vi "Replace_data_in_setup_string.vi"(1 "New data string":string, 2 "Input string":string, 3 "Variable name":string) -> (0 "Appended string":string)   [LabVIEW 2020]
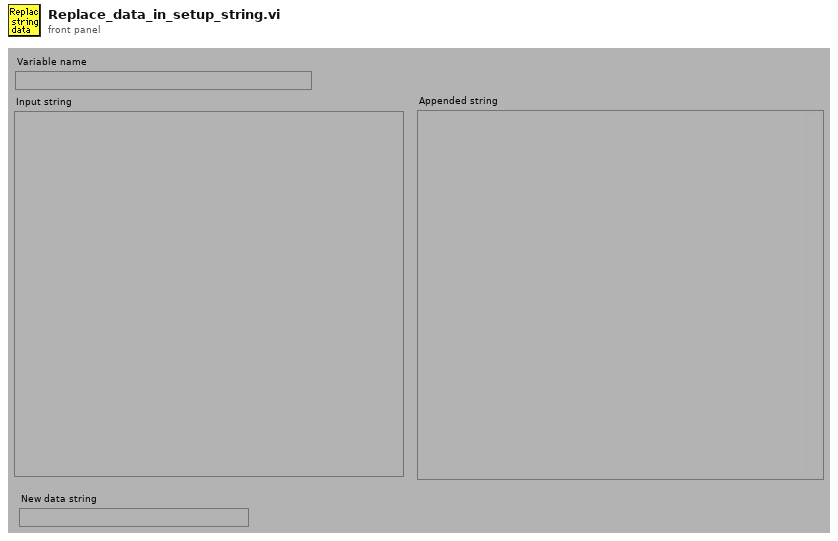
[diagram p1: front panel]
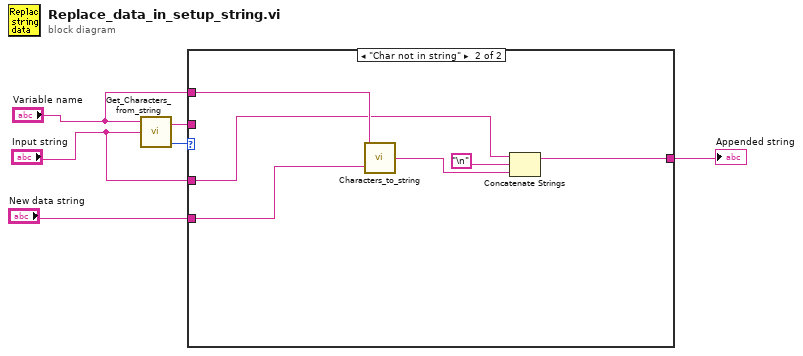
[diagram p0: block diagram]
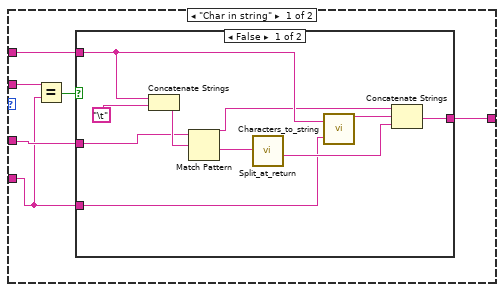
[diagram p2: hidden frame]
diagram:
  n1 = call "Get_Characters_from_string.vi"("Input string"="Input string", "Variable name"="Variable name") -> ("Status"=w6:enum16{"Char in string", "Char not in string"}, "Value"=w1:string)  [unwired: 1 in]
  n2 = case shown="\"Char not in string\"" w6 {
    tunnel: "Variable name" -> [w10 w29]
    tunnel: "New data string" -> [w8 w28]
    tunnel: [w11 w27] -> w3
    tunnel: "Input string" -> [w12 w26]
    tunnel: w1 -> [w9 _]
    frame "Char in string" {
      n3 = Equal?(x=w9, y=w8) -> (x = y?=w7:bool)
      n4 = case shown="False" w7 {
        tunnel: w12 -> [w20 w23]
        tunnel: [w17 w23] -> w11
        tunnel: w8 -> [w16 _]
        tunnel: w10 -> [w15 _]
        frame False {
          n5 = Concatenate Strings(w15, "\t") -> (w21:string)
          n6 = Match Pattern(string=w20, regular expression=w21) -> (before substring=w13:string, after substring=w19:string)  [unwired: 3 out]
          n7 = call "Split_at_return.vi"("String"=w19) -> ("after substring"=w18:string)  [unwired: 1 in, 3 out]
          n8 = call "Characters_to_string.vi"("Characters to write"=w16, "Label for characters"=w15) -> ("Output string"=w14:string)  [unwired: 1 in]
          n9 = Concatenate Strings(w13, w14, w18) -> (w17:string)
        }
        frame True {
        }
      }
    }
    frame "Char not in string" {
      n10 = call "Characters_to_string.vi"("Characters to write"=w28, "Label for characters"=w29) -> ("Output string"=w25:string)  [unwired: 1 in]
      n11 = Concatenate Strings(w26, "\n", w25) -> (w27:string)
    }
  }
  "Appended string" <- w3
